vi "CopyFilesToNAS.vi"(8 "error in":errorcluster, 9 "StoreThisManyLogFilesLocally":i32=10, 10 "Config.FP_User.Paths.NAS path":path, 11 "LocalLogFolder":path) -> (0 "error out":errorcluster)   [LabVIEW 2018]
panel:
  out "Delete":string[](array[string])
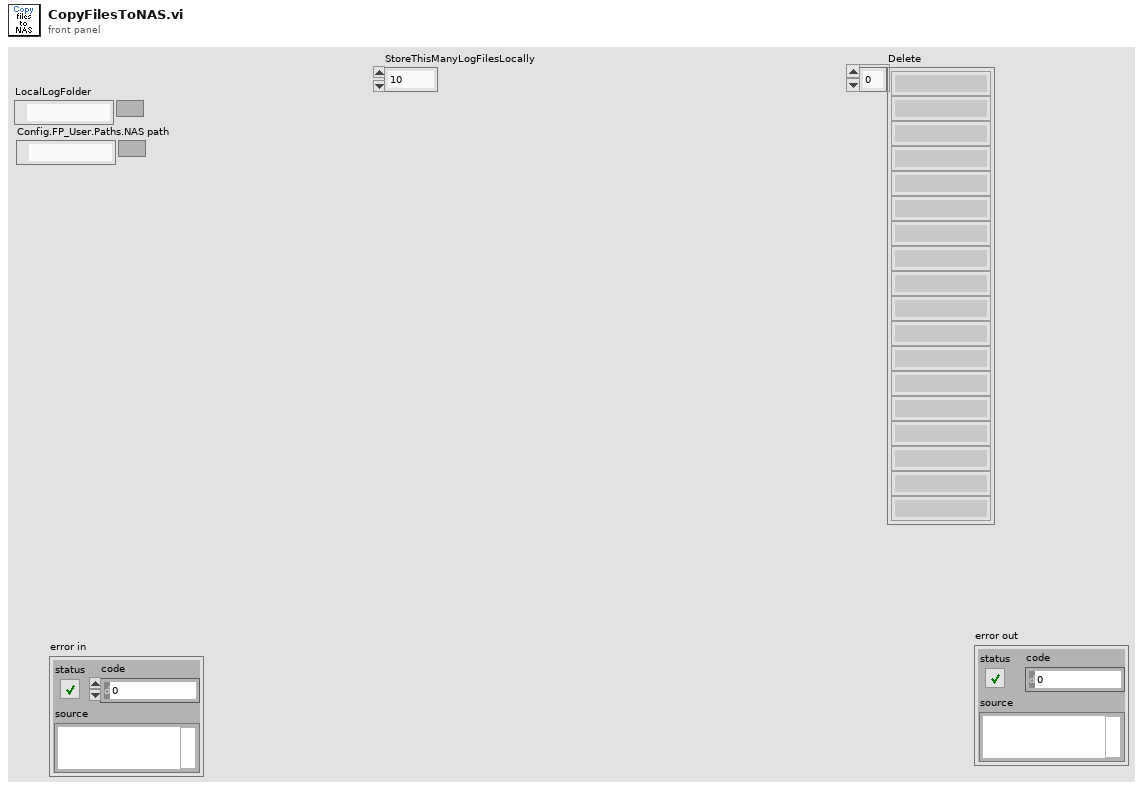
[diagram p1: front panel]
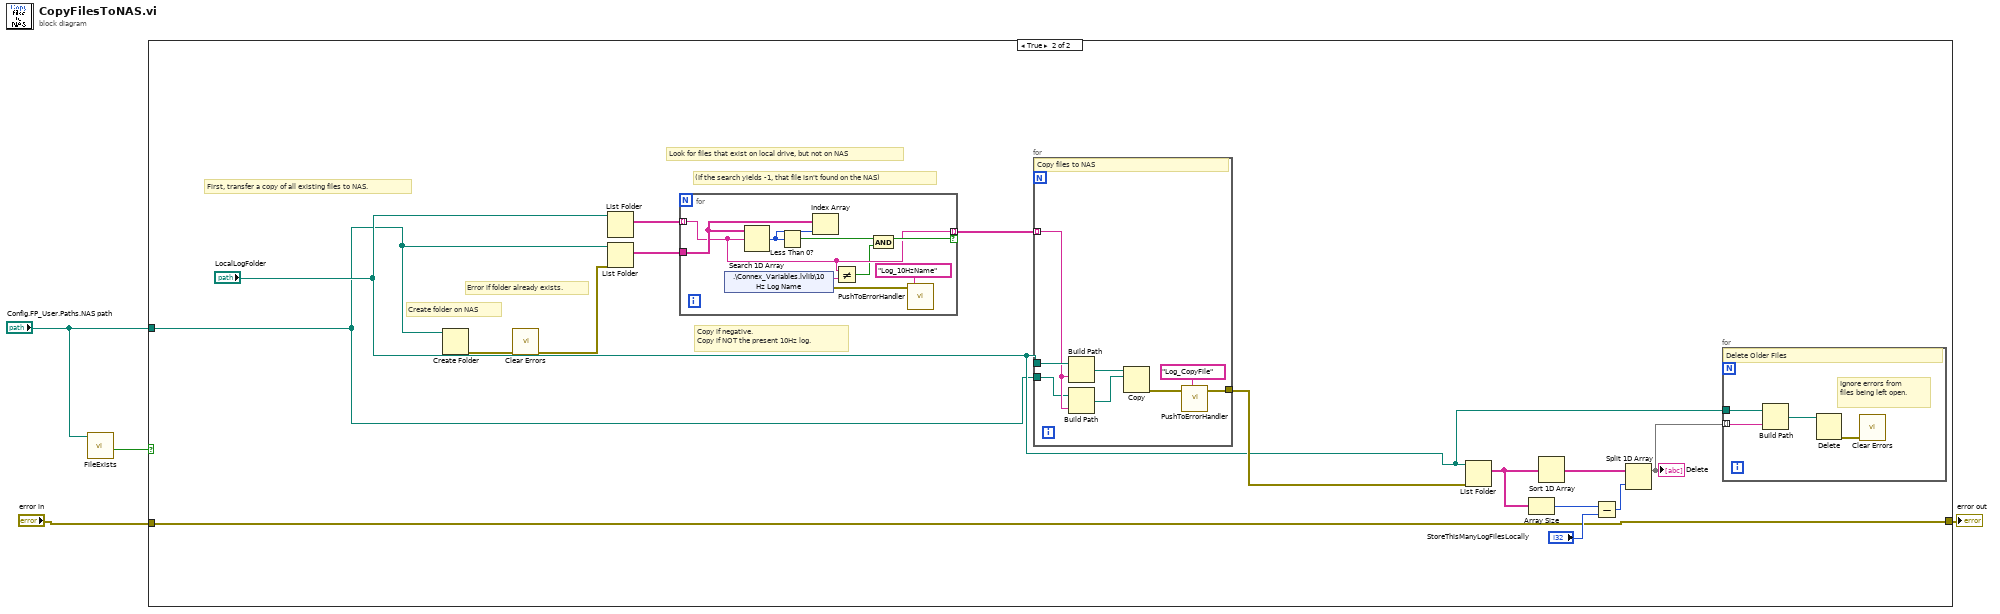
[diagram p0: block diagram]
diagram:
  n1 = call "FileExists.vi"("NAS path"="Config.FP_User.Paths.NAS path") -> ("Exists?"=w1:bool)  [unwired: 9 in, 1 out]
  n2 = case shown="True" w1 {
    tunnel: [w5 w6] -> w4
    tunnel: "Config.FP_User.Paths.NAS path" -> [_ w7]
    tunnel: "error in" -> [w5 w6]
    frame False {
      # "If NAS isn't connected, don't try to copy files.\n\nLuke"
    }
    frame True {
      # "Copy if negative.\nCopy if NOT the present 10Hz log."
      # "Create folder on NAS"
      # "Error if folder already exists."
      # "(If the search yields -1, that file isn't found on the NAS)"
      # "Look for files that exist on local drive, but not on NAS"
      # "First, transfer a copy of all existing files to NAS."
      n3 = Create Folder(path (use dialog)=w7) -> (error out=w11:errorcluster)  [unwired: 2 in, 2 out]
      n4 = call <vilib>:"Clear Errors.vi"("error in (no error)"=w11) -> ("error out"=w10:errorcluster)  [unwired: 5 in, 1 out]
      n5 = List Folder(path="LocalLogFolder") -> (filenames=w18:string[])  [unwired: 3 in, 3 out]
      n6 = List Folder(path=w7, error in=w10) -> (filenames=w19:string[])  [unwired: 2 in, 3 out]
      n7 = for {
        tunnel: w18 -> [w33] mode=indexing
        tunnel: w19 -> [w37]
        tunnel: [w33] -> w20 mode=indexing if=w34
        n8 = shared-variable ".\\Connex_Variables.lvlib\\10 Hz Log Name"() -> (w31:string, error out=w30:errorcluster)  [unwired: 1 in]
        n9 = Search 1D Array(1D array=w37, element=w33) -> (index of element=w36:i32)  [unwired: 1 in]
        n10 = Less Than 0?(x=w36) -> (x < 0?=w35:bool)
        n11 = Index Array(array=w37, index=w36) -> ()  [unwired: 1 out]
        n12 = Not Equal?(x=w33, y=w31) -> (x != y?=w32:bool)
        n13 = And(x=w35, y=w32) -> (x .and. y?=w34:bool)
        n14 = call "PushToErrorHandler.vi"("ErrorIn"=w30, "ErrorLocation"="Log_10HzName") -> ()  [unwired: 5 in, 1 out]
      }
      n15 = for {
        tunnel: "LocalLogFolder" -> [w28]
        tunnel: w7 -> [w26]
        tunnel: w20 -> [w27] mode=indexing
        tunnel: [w21] -> w9
        # "Copy files to NAS"
        n16 = Build Path(base path=w28, name or relative path=w27) -> (appended path=w25:path)
        n17 = Build Path(base path=w26, name or relative path=w27) -> (appended path=w24:path)
        n18 = Copy(10:w24, 11:w25) -> (0:w23:errorcluster)  [unwired: 3 in, 2 out]
        n19 = call "PushToErrorHandler.vi"("ErrorIn"=w23, "ErrorLocation"="Log_CopyFile") -> ("ErrorOut"=w21:errorcluster)  [unwired: 5 in]
      }
      n20 = List Folder(path="LocalLogFolder", error in=w9) -> (filenames=w16:string[])  [unwired: 2 in, 3 out]
      n21 = Array Size(array=w16) -> (size(s)=w15:i32)
      n22 = Sort 1D Array(array=w16) -> (sorted array=w17:string[])
      n23 = Subtract(x=w15, y="StoreThisManyLogFilesLocally") -> (x-y=w13:i32)
      n24 = Split 1D Array(array=w17, index=w13) -> (first subarray=w12:string[])  [unwired: 1 out]
      "Delete" <- w12
      n25 = for {
        tunnel: "LocalLogFolder" -> [w41]
        tunnel: w12 -> [w40] mode=indexing
        # "Ignore errors from files being left open."
        # "Delete Older Files"
        n26 = Build Path(base path=w41, name or relative path=w40) -> (appended path=w39:path)
        n27 = Delete(path (use dialog)=w39) -> (error out=w38:errorcluster)  [unwired: 4 in, 2 out]
        n28 = call <vilib>:"Clear Errors.vi"("error in (no error)"=w38) -> ()  [unwired: 5 in, 2 out]
      }
    }
  }
  "error out" <- w4
